vi "Unpack For Grpc.vi"(8 "error in (no error)":errorcluster, 9 "Configuration / Resuls (Config)":enum16{"Configuration", "Results"}(ring), 10 "Any":T1, 11 "Measurement Customizations in":refnum<class "MeasurementPlugin.lvclass">) -> (0 "error out":errorcluster, 2 "Data Value":variant, 3 "Measurement Customizations out":refnum<class "MeasurementPlugin.lvclass">)   [LabVIEW 2021, in "audio_acMeasurement.lvlib" / "MeasurementPlugin.lvclass"]
uses:
  MeasurementPlugin.lvclass
  <vilib>/gRPC/LabVIEW gRPC Library/Shared/Any.ctl
  Measurement Configuration.ctl
  Measurement Results.ctl
  a521b266-ce99-437c-923d-067dcf1e07fd.vi
  3ecd018e-d556-4cbc-bc60-c4ba57204520.vi
  <vilib>/gRPC/LabVIEW gRPC Library/Server API/Translate Protobuf Error.vi
  <vilib>/AdvancedString/1D String Array to Delimited String.vi
  <vilib>/gRPC/LabVIEW gRPC Library/Server API/Server/Get Server DLL Path.vi
  audio_acMeasurement.lvlib
  <vilib>/gRPC/LabVIEW gRPC Library/grpc-lvsupport-release.lvlib
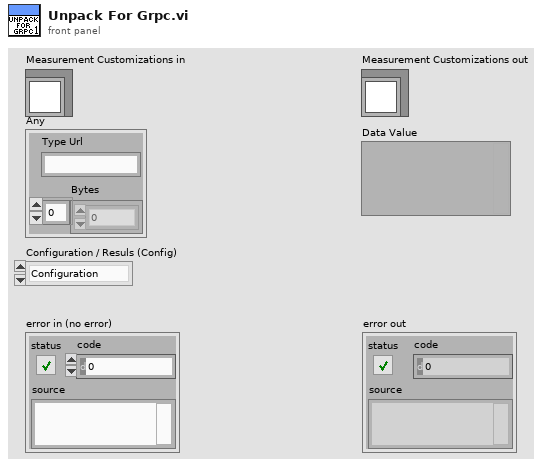
[diagram p1: front panel]
types:
  T1 = typedef "grpc-lvsupport-release.lvlib/Any.ctl" = cluster{"Type Url":string, "Bytes":u8[]}
  T2 = typedef "grpc-lvsupport-release.lvlib/grpcId.ctl" = u64
  T3 = typedef "audio_acMeasurement.lvlib/Measurement Configuration.ctl" = cluster{"Band start":dbl, "Band stop":dbl, "Weighting filter":u16, "Full scale range":dbl, "Analog source resource name":string, "Frequency":dbl, "Amplitude":dbl, "Protocol capture resource name":string, "Protocol":string, "Clock rate":u32, "Number of words":i32, "Sensitivity":dbl}
  T4 = typedef "audio_acMeasurement.lvlib/Measurement Results.ctl" = cluster{"Channel":string, "Calculated frequency":dbl, "Calculated amplitude":dbl, "SNR":dbl, "THD+N":dbl, "THD":dbl, "Dynamic range":dbl, "Gain error":dbl, "SFDR":dbl, "t0":dbl, "dt":dbl, "Time domain":dbl[], "f0":dbl, "df":dbl, "Spectrum":dbl[], "Calculated sample rate":u32}
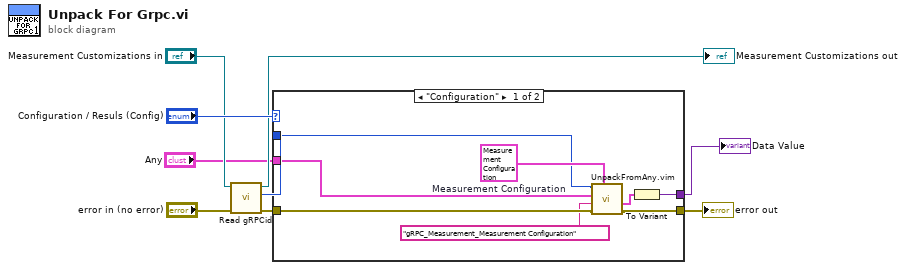
[diagram p0: block diagram]
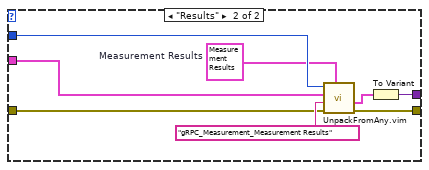
[diagram p2: hidden frame]
diagram:
  n1 = call-dynamic "Read gRPCid.vi"("error in"="error in (no error)", "iService in"="Measurement Customizations in") -> ("error out"=w6:errorcluster, "gRPCid"=w3:T2, "iService out"=→"Measurement Customizations out":refnum<class "MeasurementPlugin.lvclass">)  [unwired: 7 in]
  n2 = case shown="\"Configuration\"" "Configuration / Resuls (Config)" {
    tunnel: w6 -> [w15 w19]
    tunnel: "Any" -> [w10 w18]
    tunnel: w3 -> [w12 w22]
    tunnel: [w16 w23] -> w9
    tunnel: [w17 w25] -> w1
    frame "Configuration" {
      w13 = T3 {"Band start"=20.0, "Band stop"=20000.0, "Weighting filter"=0, "Full scale range"=3.16, "Analog source resource name"="", "Frequency"=1000.0, "Amplitude"=1.0, "Protocol capture resource name"="PXI1Slot7\\I2Si 0", "Protocol"="", "Clock rate"=12288000, "Number of words"=19200, "Sensitivity"=0.34762}  # Measurement Configuration
      n3 = call "UnpackFromAny.vim"("Data Type"=w13, "error in"=w15, "Message Type"="gRPC_Measurement_Measurement Configuration", "Any"=w10, "gRPCid in"=w12) -> ("error out"=w16:errorcluster, "Unpacked Value"=w14:T3)  [unwired: 4 in, 1 out]
      n4 = To Variant(anything=w14) -> (Variant=w17:variant)
    }
    frame "Results" {
      w21 = T4 {"Channel"="", "Calculated frequency"=0.0, "Calculated amplitude"=0.0, "SNR"=0.0, "THD+N"=0.0, "THD"=0.0, "Dynamic range"=0.0, "Gain error"=0.0, "SFDR"=0.0, "t0"=0.0, "dt"=0.0, "Time domain"=[], "f0"=0.0, "df"=0.0, "Spectrum"=[], "Calculated sample rate"=0}  # Measurement Results
      n5 = call "UnpackFromAny.vim"("Data Type"=w21, "error in"=w19, "Message Type"="gRPC_Measurement_Measurement Results", "Any"=w18, "gRPCid in"=w22) -> ("error out"=w23:errorcluster, "Unpacked Value"=w24:T4)  [unwired: 4 in, 1 out]
      n6 = To Variant(anything=w24) -> (Variant=w25:variant)
    }
  }
  "error out" <- w9
  "Data Value" <- w1
